vi "Post-Uninstall Custom Action.vi"(10 "Variant":variant) -> (0 "error out":errorcluster)   [LabVIEW 2020]
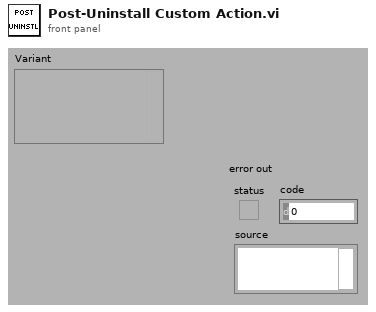
[diagram p1: front panel]
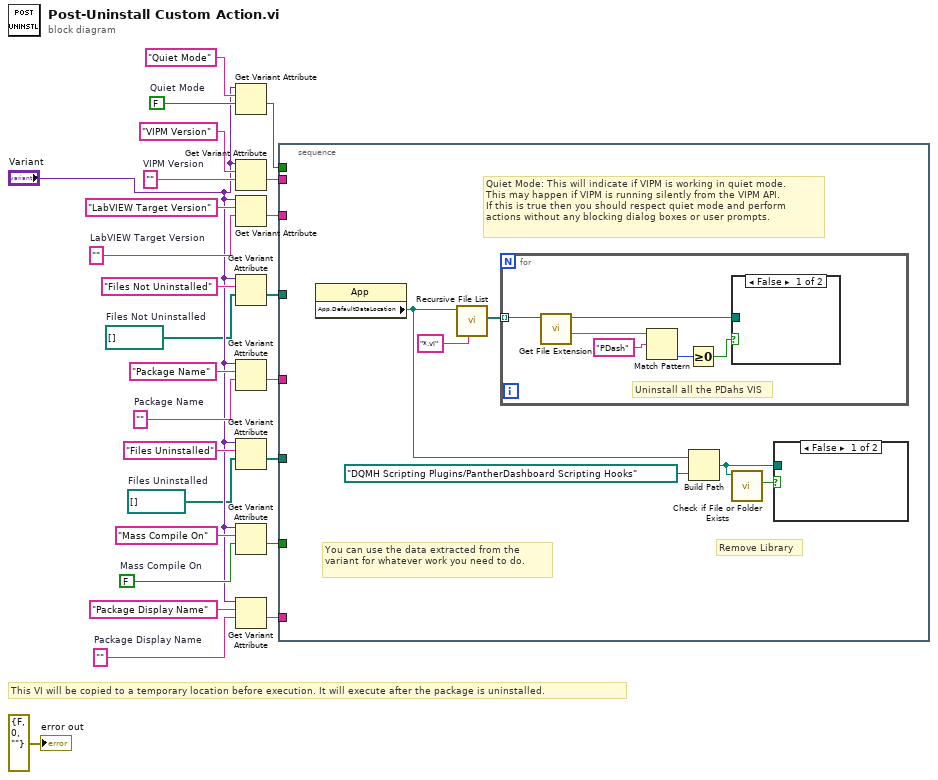
[diagram p0: block diagram]
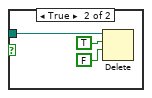
[diagram p2: hidden frame]
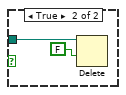
[diagram p3: hidden frame]
diagram:
  w1 = path[] []  # Files Not Uninstalled
  w2 = path[] []  # Files Uninstalled
  w8 = FALSE  # Mass Compile On
  w9 = ""  # Package Display Name
  w16 = FALSE  # Quiet Mode
  w19 = ""  # VIPM Version
  w21 = ""  # LabVIEW Target Version
  w23 = ""  # Package Name
  # "This VI will be copied to a temporary location before execution. It will execute after the package is uninstalled."
  n1 = Get Variant Attribute(Variant="Variant", name="Quiet Mode", default value (empty Variant)=w16) -> (value=w11:bool)  [unwired: 1 in, 3 out]
  n2 = Get Variant Attribute(Variant="Variant", name="VIPM Version", default value (empty Variant)=w19) -> (value=w12:string)  [unwired: 1 in, 3 out]
  n3 = Get Variant Attribute(Variant="Variant", name="LabVIEW Target Version", default value (empty Variant)=w21) -> (value=w13:string)  [unwired: 1 in, 3 out]
  n4 = Get Variant Attribute(Variant="Variant", name="Files Not Uninstalled", default value (empty Variant)=w1) -> (value=w6:path[])  [unwired: 1 in, 3 out]
  n5 = Get Variant Attribute(Variant="Variant", name="Package Name", default value (empty Variant)=w23) -> (value=w14:string)  [unwired: 1 in, 3 out]
  n6 = Get Variant Attribute(Variant="Variant", name="Files Uninstalled", default value (empty Variant)=w2) -> (value=w5:path[])  [unwired: 1 in, 3 out]
  n7 = Get Variant Attribute(Variant="Variant", name="Mass Compile On", default value (empty Variant)=w8) -> (value=w10:bool)  [unwired: 1 in, 3 out]
  n8 = Get Variant Attribute(Variant="Variant", name="Package Display Name", default value (empty Variant)=w9) -> (value=w15:string)  [unwired: 1 in, 3 out]
  n9 = stacked-sequence {
    tunnel: w15 -> [_]
    tunnel: w14 -> [_]
    tunnel: w13 -> [_]
    tunnel: w12 -> [_]
    tunnel: w11 -> [_]
    tunnel: w10 -> [_]
    tunnel: w5 -> [_]
    tunnel: w6 -> [_]
    frame #0 {
      # "Remove Library"
      # "Quiet Mode: This will indicate if VIPM is working in quiet mode.\nThis may happen if VIPM is running silently from the VIPM API.\nIf this is true then you should respect quiet mode and perform\nactions without any blocking dialog boxes or user prompts."
      # "You can use the data extracted from the variant for whatever work you need to do."
      n10 = property class="App"() -> ("App.DefaultDataLocation"=w31:path)  [unwired: 2 in, 2 out]
      n11 = call <vilib>:"Recursive File List.vi"("pattern"="*.vi", "Folder Path"=w31) -> ("All Files in Dir"=w32:path[])  [unwired: 5 in, 4 out]
      n12 = for {
        tunnel: w32 -> [w41] mode=indexing
        # "Uninstall all the PDahs VIS"
        n13 = call <vilib>:"Get File Extension.vi"("file"=w41) -> ("filename without extension"=w40:string, "dup file"=w37:path)  [unwired: 6 in, 3 out]
        n14 = Match Pattern(string=w40, regular expression="PDash") -> (offset past match=w38:i32)  [unwired: 1 in, 3 out]
        n15 = Greater Or Equal To 0?(x=w38) -> (x >= 0?=w36:bool)
        n16 = case shown="False" w36 {
          tunnel: w37 -> [_ w43]
          frame False {
          }
          frame True {
            n17 = Delete(path (use dialog)=w43, confirm (F)=FALSE) -> ()  [unwired: 3 in, 3 out]
          }
        }
      }
      n18 = Build Path(base path=w31, name or relative path=path "DQMH Scripting Plugins/PantherDashboard Scripting Hooks") -> (appended path=w29:path)
      n19 = call <vilib>:"Check if File or Folder Exists.vi"("path"=w29) -> ("file or folder exists?"=w28:bool)  [unwired: 8 in, 2 out]
      n20 = case shown="False" w28 {
        tunnel: w29 -> [_ w35]
        frame False {
        }
        frame True {
          n21 = Delete(path (use dialog)=w35, entire hierarchy (F)=TRUE, confirm (F)=FALSE) -> ()  [unwired: 2 in, 3 out]
        }
      }
    }
  }
  "error out" <- errorcluster {"status"=FALSE, "code"=0, "source"=""} ("error out")
